vi "Arm Hardware.vi"(8 "error in (no error)":errorcluster, 9 "Request type":T1=enum."User command", 11 "Micron sm Digitizer in":refnum<class "Micron sm Digitizer.lvclass">) -> (0 "error out":errorcluster, 3 "Micron sm Digitizer out":refnum<class "Micron sm Digitizer.lvclass">)   [LabVIEW 2024, in "Micron sm Digitizer.lvclass"]
uses:
  Micron sm Digitizer.lvclass
  LabActor/Controllers/Process Controller/Request type.ctl
  VISA Instrument/VISA Instrument.lvclass/VISA Instrument.ctl
  Instrument Driver/Instrument Driver.lvclass/Instrument Driver.ctl
  Micron sm Digitizer.lvclass/Micron sm Digitizer.ctl
  Pulse Driver/Pulse Driver.lvclass/Pulse Driver.ctl
  VISA Instrument/Read VISA resource.vi
  Instrument Driver/Read Recorder name.vi
  VISA Instrument/Write VISA resource.vi
  Write Latch trigger.vi
  Pulse Driver/Write dt.vi
  Pulse Driver/Write t0.vi
  Micron Optics Driver/Micron Optics Driver.lvclass
  Micron Optics sm130/Micron Optics sm130.lvlib
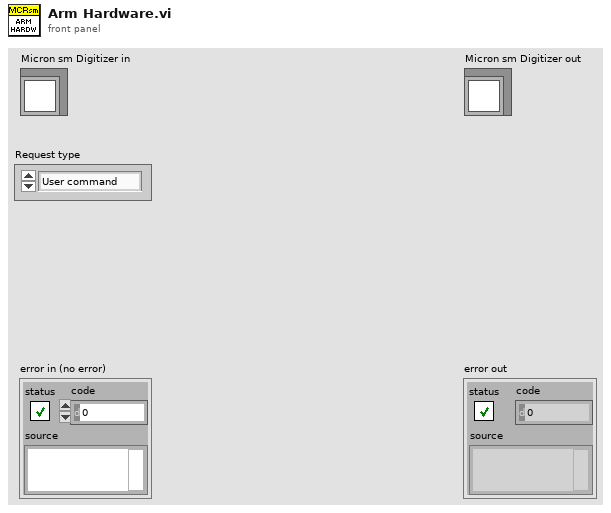
[diagram p1: front panel]
types:
  T1 = typedef "Request type.ctl" = enum16{"Process complete", "User command", "Auto-restart", "Error"}
  T2 = typedef "Micron optics didgitizer configuration.ctl" = cluster{"Post-trigger delay":dbl, "Post-trigger duration":dbl, "Rate":dbl, "Reference channel":i32, "Detection Setting IDs":u8[], "Stream and average":bool, "Address":string}
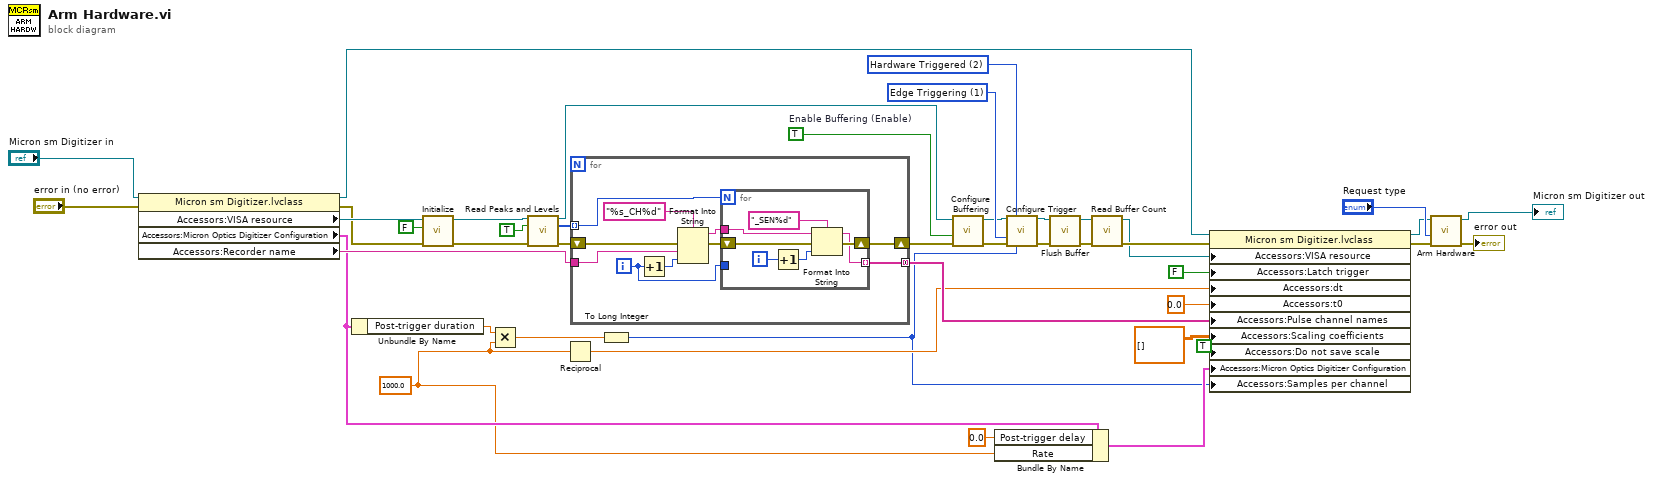
[diagram p0: block diagram]
diagram:
  w2 = 1000.0
  w25 = TRUE  # Enable Buffering (Enable)
  w36 = u16 1 items=["Number of Acquisitions", "Edge Triggering"] ("Trigger Stop Condition (1:Edge Triggering)")
  w37 = u16 2 items=["Untriggered", "Software Triggered", "Hardware Triggered"] ("Trigger Type (0:Untriggered)")
  n1 = property class="Micron sm Digitizer.lvclass"(reference="Micron sm Digitizer in", error in="error in (no error)") -> (reference out=w32:refnum<class "Micron sm Digitizer.lvclass">, error out=w7:errorcluster, "Accessors:VISA resource"=w38:refnum<visa-resource-name>, "Accessors:Micron Optics Digitizer Configuration"=w5:T2, "Accessors:Recorder name"=w14:string)
  n2 = Unbundle By Name(w5) -> ("Post-trigger duration"=w35:dbl)
  n3 = call "Initialize.vi"("error in (no error)"=w7, "ID Query (True)"=FALSE, "VISA resource name"=w38) -> ("error out"=w19:errorcluster, "VISA resource name out"=w18:refnum<visa-resource-name>)  [unwired: 7 in]
  n4 = Multiply(x=w35, y=w2) -> (x*y=w34:dbl)
  n5 = call "Read Peaks and Levels.vi"("VISA resource name"=w18, "Enable Unbuffered Data (Enabled)"=TRUE, "error in (no error)"=w19) -> ("VISA resource name out"=w17:refnum<visa-resource-name>, "Number of Sensors"=w15:u16[], "error out"=w13:errorcluster)  [unwired: 4 in, 6 out]
  n6 = Reciprocal(x=w2) -> (1/x=w8:dbl)
  n7 = for {
    tunnel: w15 -> [w53] mode=indexing
    tunnel: w14 -> [w51]
    shift-right: [w46] -> w12
    shift-left: w13 -> [w48]
    tunnel: [w44] -> w11 mode=concatenating
    i -> [w45]
    n8 = Increment(x=w45) -> (x+1=w50:i32)
    n9 = Format Into String(format string="%s_CH%d", error in=w48, w51, w50) -> (resulting string=w49:string, error out=w47:errorcluster)  [unwired: 1 in]
    n10 = for {
      N: w53 -> [_]
      tunnel: w49 -> [w60]
      shift-right: [w55] -> w46
      shift-left: w47 -> [w58]
      tunnel: w45 -> [_]
      tunnel: [w54] -> w44 mode=indexing
      i -> [w56]
      n11 = Increment(x=w56) -> (x+1=w57:i32)
      n12 = Format Into String(format string="_SEN%d", initial string=w60, error in=w58, w57) -> (resulting string=w54:string, error out=w55:errorcluster)
    }
  }
  n13 = To Long Integer(number=w34) -> (32bit integer=w1:i32)
  n14 = call "Configure Buffering.vi"("error in (no error)"=w12, "Enable Buffering (Enable)"=w25, "VISA resource name"=w17) -> ("error out"=w26:errorcluster, "VISA resource name out"=w27:refnum<visa-resource-name>)  [unwired: 6 in, 1 out]
  n15 = Bundle By Name(cluster=w5, "Post-trigger delay"=0.0, "Rate"=w2) -> (w3:T2)
  n16 = call "Configure Trigger.vi"("VISA resource name"=w27, "Trigger Type (0:Untriggered)"=w37, "Trigger Stop Condition (1:Edge Triggering)"=w36, "error in (no error)"=w26, "Number of Acquisitions (100)"=w1) -> ("VISA resource name out"=w22:refnum<visa-resource-name>, "error out"=w21:errorcluster)  [unwired: 8 in, 1 out]
  n17 = call "Flush Buffer.vi"("error in (no error)"=w21, "VISA resource name"=w22) -> ("error out"=w28:errorcluster, "VISA resource name out"=w29:refnum<visa-resource-name>)  [unwired: 8 in]
  n18 = call "Read Buffer Count.vi"("error in"=w28, "VISA resource name"=w29) -> ("error out"=w24:errorcluster, "VISA resource name out"=w23:refnum<visa-resource-name>)  [unwired: 6 in, 2 out]
  n19 = property class="Micron sm Digitizer.lvclass"(reference=w32, error in=w24, "Accessors:VISA resource"=w23, "Accessors:Latch trigger"=FALSE ("Latch trigger"), "Accessors:dt"=w8, "Accessors:t0"=0.0 ("t0"), "Accessors:Pulse channel names"=w11, "Accessors:Scaling coefficients"=dbl[][] [] ("Scaling coefficients"), "Accessors:Do not save scale"=TRUE ("Do not save scale"), "Accessors:Micron Optics Digitizer Configuration"=w3, "Accessors:Samples per channel"=w1) -> (reference out=w33:refnum<class "Micron sm Digitizer.lvclass">, error out=w31:errorcluster)
  n20 = call-parent "Arm Hardware.vi"("error in (no error)"=w31, "Request type"="Request type", "Pulse Driver in"=w33) -> ("error out"=→"error out":errorcluster, "Pulse Driver out"=→"Micron sm Digitizer out":refnum<class "Micron sm Digitizer.lvclass">)  [unwired: 7 in]
